vi "Page_Drivers_Read.vi"(6 "ctlReferences":T1, 8 "error in (no error)":errorcluster, 11 "Class in":refnum<class "IB_MSI.lvclass">) -> (0 "error out":errorcluster, 3 "Class out":refnum<class "IB_MSI.lvclass">)   [LabVIEW 2020, in "IB_MSI.lvclass"]
uses:
  <vilib>/AppBuilder/IB_Classes/MSI/IB_MSI.lvclass
  <vilib>/AppBuilder/IB_Classes/MSI/IB_MSI.lvclass/IB_MSI.ctl
  AppLibs/distkit/MDF/NI_MDF.lvlib
  AppLibs/distkit/MDF/NIMdf.llb/MDFCommonOptions.ctl
  <resource>/Framework/Providers/Builds/Installer/Pages/controls/IB_UI_Page_Drivers_References.ctl
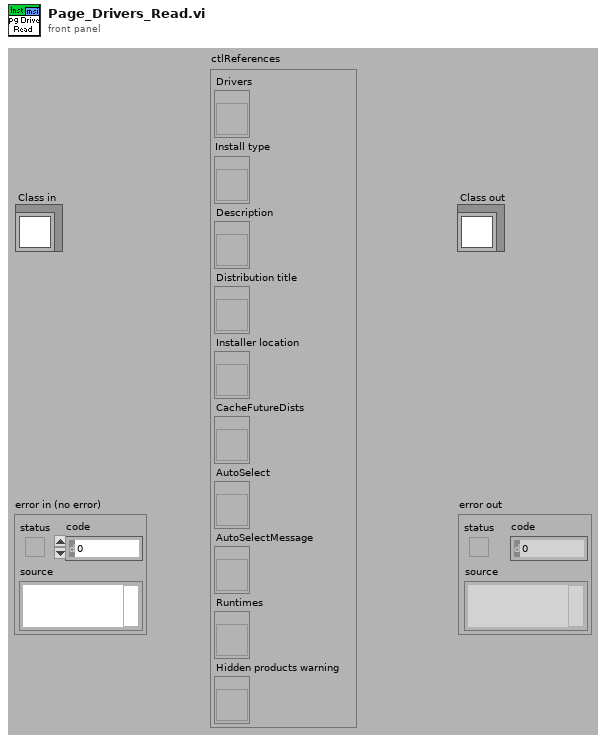
[diagram p1: front panel]
types:
  T1 = typedef "IB_UI_Page_Drivers_References.ctl" = cluster{"Drivers":refnum<vi>, "Install type":refnum<vi>, "Description":refnum<vi>, "Distribution title":refnum<vi>, "Installer location":refnum<vi>, "CacheFutureDists":refnum<vi>, "AutoSelect":refnum<vi>, "AutoSelectMessage":refnum<vi>, "Runtimes":refnum<vi>, "Hidden products warning":refnum<vi>}
  T2 = typedef "NI_MDF.lvlib/MDFCommonOptions.ctl" = i32
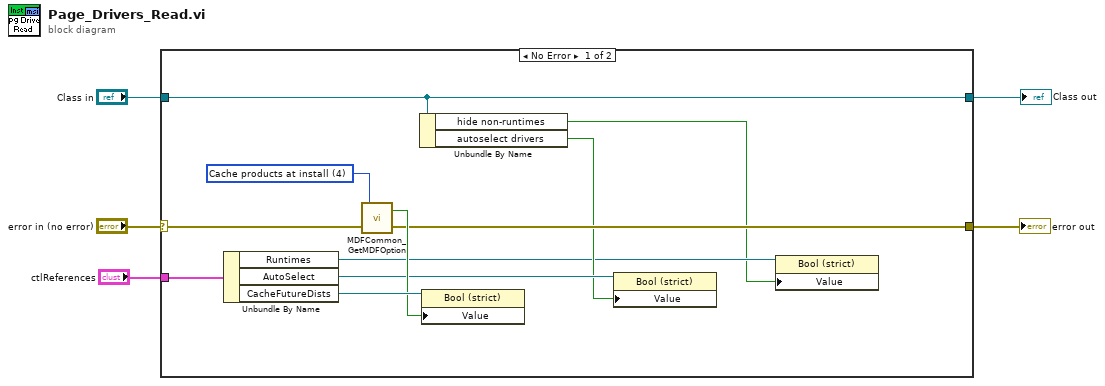
[diagram p0: block diagram]
diagram:
  n1 = case shown="No Error" "error in (no error)" {
    selector: "error in (no error)" -> [w12 w18]
    tunnel: [w13 w18] -> w4
    tunnel: "Class in" -> [w8 w17]
    tunnel: "ctlReferences" -> [w9 _]
    tunnel: [w8 w17] -> w1
    frame No Error {
      w15 = T2 4 items=["Include patch targets with patches"=1, "Cache products at disk prompt"=2, "Cache products at install"=4] ("option to get")
      n2 = Unbundle By Name(w9) -> ("Runtimes"=w7:refnum<vi>, "AutoSelect"=w11:refnum<vi>, "CacheFutureDists"=w16:refnum<vi>)
      n3 = call "MDFCommon_GetMDFOption.vi"("error in (no error)"=w12, "option to get"=w15) -> ("error out"=w13:errorcluster, "option value"=w14:bool)
      n4 = Unbundle By Name(w8) -> ("hide non-runtimes"=w6:bool, "autoselect drivers"=w10:bool)
      n5 = property class="Bool (strict)"(reference=w16, "Value"=w14) -> ()  [unwired: 1 in, 2 out]
      n6 = property class="Bool (strict)"(reference=w11, "Value"=w10) -> ()  [unwired: 1 in, 2 out]
      n7 = property class="Bool (strict)"(reference=w7, "Value"=w6) -> ()  [unwired: 1 in, 2 out]
    }
    frame Error {
    }
  }
  "error out" <- w4
  "Class out" <- w1
